vi "Recieve Theme From Caller.vi"(8 "Error In":errorcluster, 10 "Theme DVR":refnum<data-value>, 11 "Appearance Actor in":refnum<class "Appearance Actor.lvclass">) -> (0 "Error Out":errorcluster, 3 "Appearance Actor out":refnum<class "Appearance Actor.lvclass">)   [LabVIEW 2021, in "Appearance Actor.lvlib" / "Appearance Actor.lvclass"]
uses:
  Appearance Actor.lvclass
  C:/Program Files (x86)/National Instruments/LabVIEW 2021/vi.lib/ActorFramework/Actor/Actor.lvclass
  Theme Classes/Generic Theme/Generic Theme.lvclass
  Appearance Actor.lvclass/Appearance Actor.ctl
  <vilib>/ActorFramework/Actor/Actor.lvclass/Actor.ctl
  <vilib>/ActorFramework/Message Enqueuer/Message Enqueuer.lvclass/Message Enqueuer.ctl
  <vilib>/ActorFramework/Message Enqueuer/Init from Existing Queue.vi
  <vilib>/ActorFramework/Message Enqueuer/Enqueue.vi
  Appearance Actor Messages/Propagate Theme To Nested Appearance Actors Msg/Propagate Theme To Nested Appearance Actors Msg.lvclass
  C:/Program Files (x86)/National Instruments/LabVIEW 2021/vi.lib/ActorFramework/Message/Message.lvclass
  Appearance Actor Messages/Apply Theme Msg/Apply Theme Msg.lvclass
  <vilib>/ActorFramework/Message Priority Queue/Priority Enqueue.vi
  <vilib>/ActorFramework/Message Enqueuer/Message Enqueuer.lvclass
  <vilib>/ActorFramework/Actor/Actor.lvclass
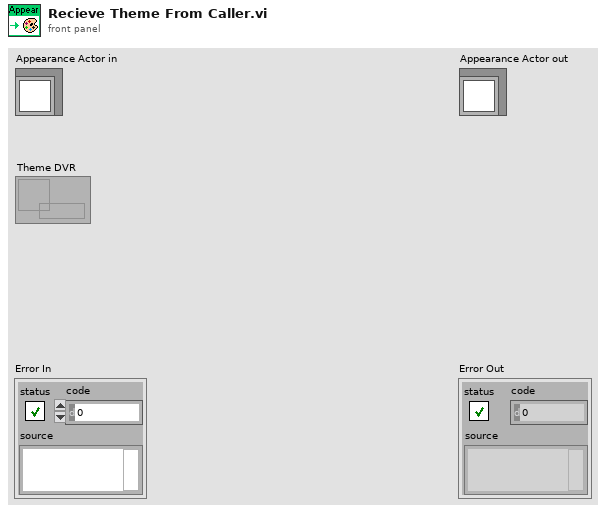
[diagram p1: front panel]
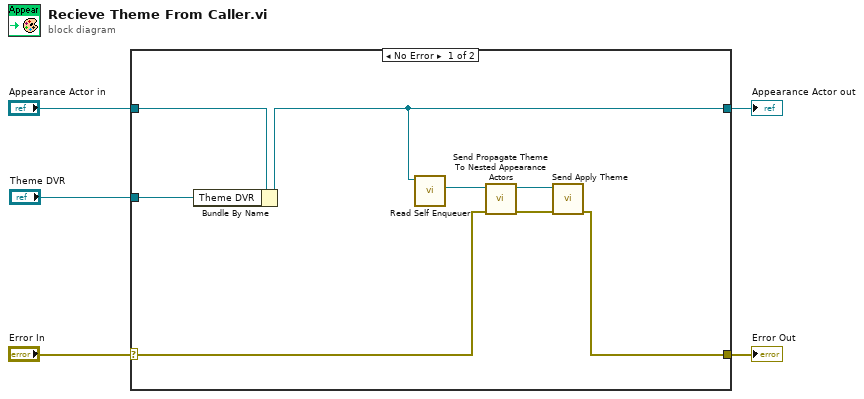
[diagram p0: block diagram]
diagram:
  n1 = case shown="No Error" "Error In" {
    selector: "Error In" -> [w8 w15]
    tunnel: [w7 w15] -> w4
    tunnel: [w9 w14] -> w2
    tunnel: "Appearance Actor in" -> [w13 w14]
    tunnel: "Theme DVR" -> [w6 _]
    frame No Error {
      n2 = Bundle By Name(cluster=w13, "Theme DVR"=w6) -> (w9:refnum<class "Appearance Actor.lvclass">)
      n3 = call <vilib>:"Read Self Enqueuer.vi"("Actor"=w9) -> ("Self Enqueuer"=w10:refnum<class "Message Enqueuer.lvclass">)  [unwired: 10 in]
      n4 = call "Send Propagate Theme To Nested Appearance Actors.vi"("error in (no error)"=w8, "Message Enqueuer"=w10) -> ("error out"=w11:errorcluster, "Message Enqueuer out"=w12:refnum<class "Message Enqueuer.lvclass">)  [unwired: 8 in]
      n5 = call "Send Apply Theme.vi"("error in (no error)"=w11, "Message Enqueuer"=w12) -> ("error out"=w7:errorcluster)  [unwired: 8 in, 1 out]
    }
    frame Error {
    }
  }
  "Error Out" <- w4
  "Appearance Actor out" <- w2
